vi "Write Snake DVR.vi"(8 "error in (no error)":errorcluster, 10 "Board Game in":refnum<class "Board Game.lvclass">, 11 "data value reference":refnum<data-value>) -> (0 "error out":errorcluster)   [LabVIEW 2021, in "Board Game.lvclass"]
uses:
  Board Game.lvclass
  Board Game.lvclass/Board Game.ctl
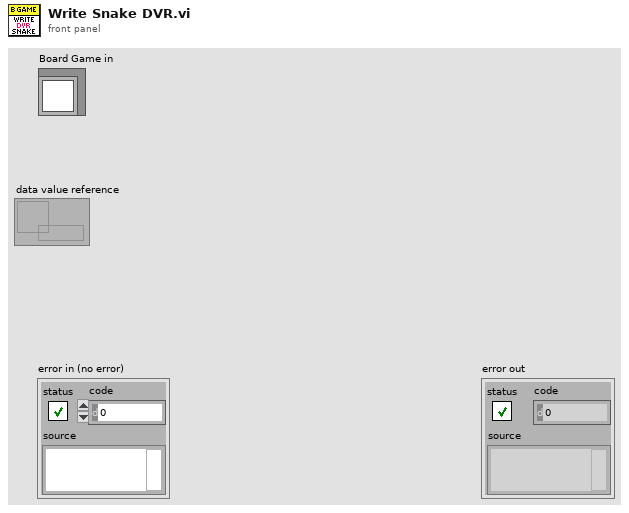
[diagram p1: front panel]
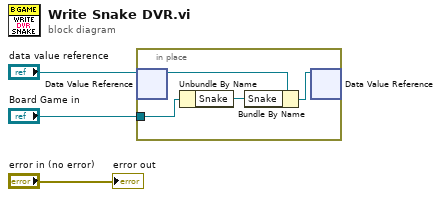
[diagram p0: block diagram]
diagram:
  n1 = in-place {
    in-place-border: "Board Game in" -> [w6]
    n2 = in-place-dvr #1("data value reference") -> (w7:refnum<class "Board Game.lvclass">)  [unwired: 1 out]
    n3 = Unbundle By Name(w6) -> ("Snake"=w4:refnum<class "Snake.lvclass">)
    n4 = Bundle By Name(cluster=w7, "Snake"=w4) -> (w5:refnum<class "Board Game.lvclass">)
    n5 = in-place-dvr #1(w5) -> ()  [unwired: 2 out]
  }
  "error out" <- "error in (no error)"
